vi "Draw Collapsed Terminals.vi"(6 "State":T7, 7 "Sizes":T6, 9 "Collapsed Types":T1[](array[typedef]), 11 "Picture  In":picture) -> (3 "Picture":picture)   [LabVIEW 2020, in "FlexBlock.xnode"]
uses:
  FlexBlock.xnode
  State.ctl
  FlexBlocks/Type Descriptor.ctl
  FlexBlocks/Terminal Direction.ctl
  FlexBlocks/Value Mode.ctl
  FlexBlocks/Terminal State.ctl
  FlexBlocks/Special Terminal.ctl
  FlexBlocks/Errors.ctl
  <vilib>/picture/picture.llb/imagedata.ctl
  FlexBlocks/Calculated Sizes.ctl
  FlexBlocks/Size Constants.ctl
  FlexBlocks/FlexBlocks.lvlib
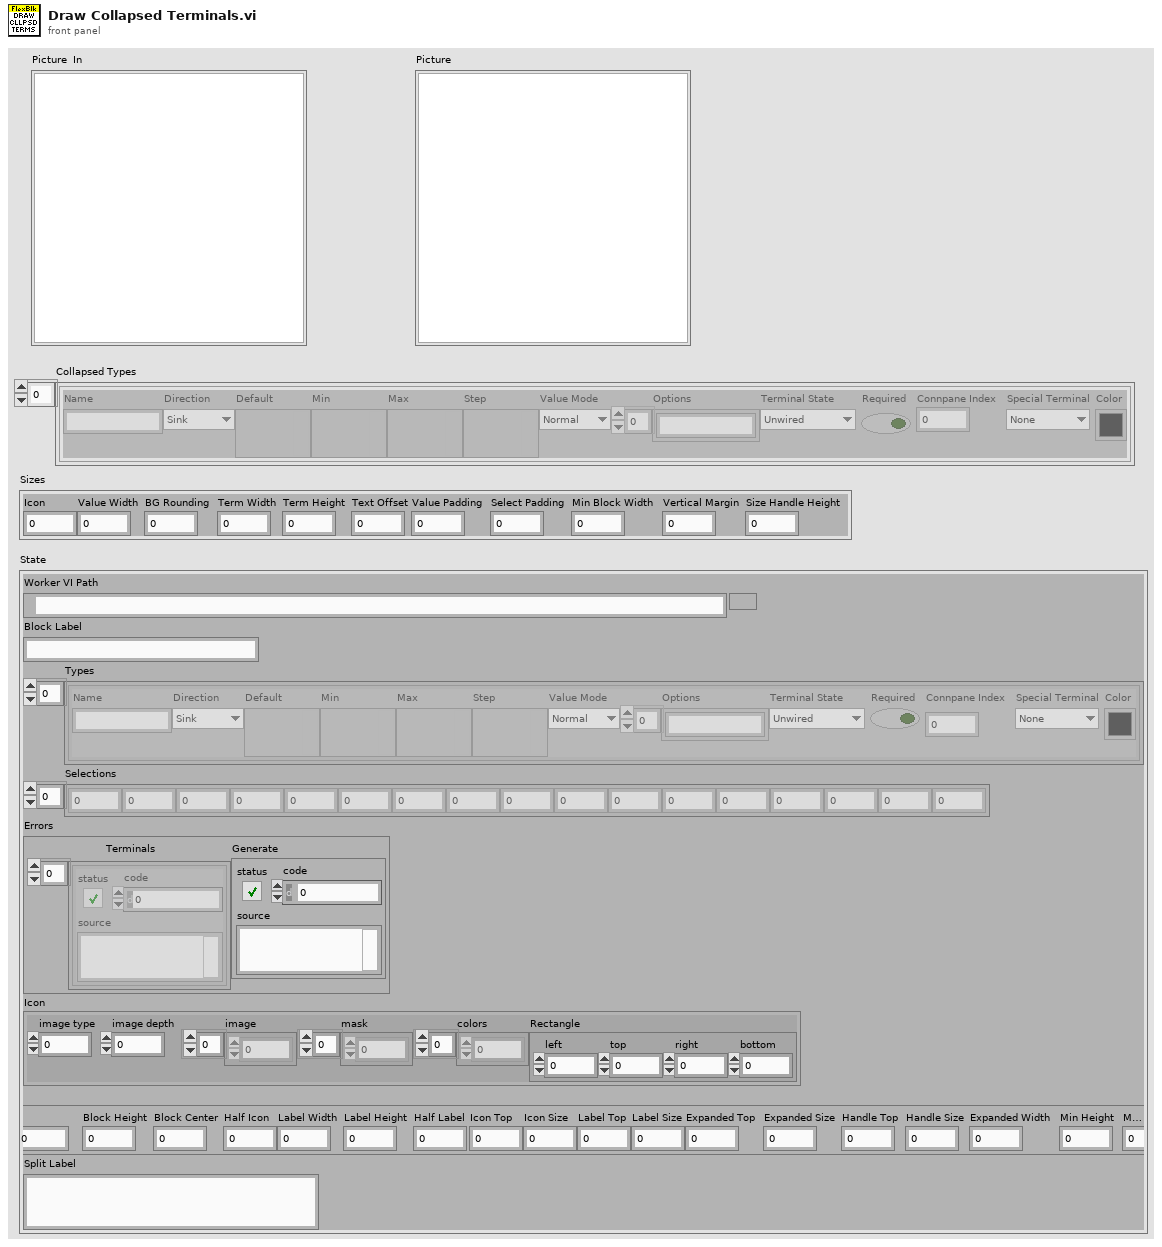
[diagram p1: front panel]
types:
  T1 = typedef "FlexBlocks.lvlib/Type Descriptor.ctl" = cluster{"Name":string, "Direction":T2, "Default":variant, "Min":variant, "Max":variant, "Step":variant, "Value Mode":T3, "Options":string[], "Terminal State":T4, "Required":bool, "Connpane Index":i32, "Special Terminal":T5, "Color":u32}
  T2 = typedef "FlexBlocks.lvlib/Terminal Direction.ctl" = enum16{"Sink", "Source"}
  T3 = typedef "FlexBlocks.lvlib/Value Mode.ctl" = enum16{"Normal", "Range", "Select"}
  T4 = typedef "FlexBlocks.lvlib/Terminal State.ctl" = enum16{"Unwired", "BadType", "BadRef", "Channel", "Value", "Control Ref"}
  T5 = typedef "FlexBlocks.lvlib/Special Terminal.ctl" = enum16{"None", "Action", "Init", "Tag", "State in", "State out", "Error"}
  T6 = typedef "FlexBlocks.lvlib/Size Constants.ctl" = cluster{"Icon":i32, "Value Width":i32, "BG Rounding":i32, "Term Width":i32, "Term Height":i32, "Text Offset":i32, "Value Padding":i32, "Select Padding":i32, "Min Block Width":i32, "Vertical Margin":i32, "Size Handle Height":i32}
  T7 = typedef "FlexBlock.xnode/State.ctl" = cluster{"Worker VI Path":path, "Block Label":string, "Types":T1[], "Selections":i32[], "Errors":T8, "Icon":T9, "Calcd Sizes":T10, "Split Label":string}
  T8 = typedef "FlexBlocks.lvlib/Errors.ctl" = cluster{"Terminals":errorcluster[], "Generate":errorcluster}
  T9 = typedef "imagedata.ctl" = cluster{"image type":i32, "image depth":i32, "image":u8[], "mask":u8[], "colors":u32[], "Rectangle":cluster{"left":i16, "top":i16, "right":i16, "bottom":i16}}
  T10 = typedef "FlexBlocks.lvlib/Calculated Sizes.ctl" = cluster{"Text Width":i32, "Text Height":i32, "Half Text":i32, "Block Width":i32, "Block Height":i32, "Block Center":i32, "Half Icon":i32, "Label Width":i32, "Label Height":i32, "Half Label":i32, "Icon Top":i32, "Icon Size":i32, "Label Top":i32, "Label Size":i32, "Expanded Top":i32, "Expanded Size":i32, "Handle Top":i32, "Handle Size":i32, "Expanded Width":i32, "Min Height":i32, "Max Height":i32}
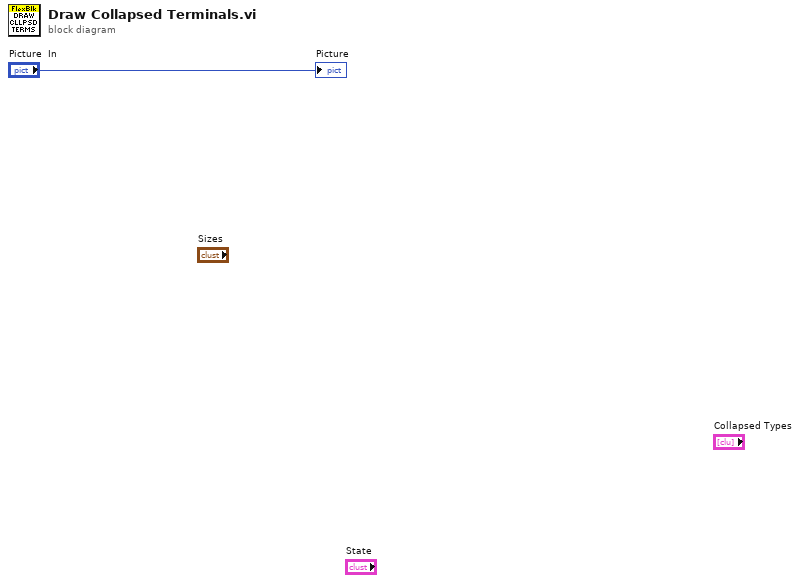
[diagram p0: block diagram]
diagram:
  "Picture" <- "Picture  In"
